vi "HandleStopAsync.vi"(8 "error in (no error)":errorcluster, 11 "S4GUI in":refnum<class "S4GUI.lvclass">) -> (0 "error out":errorcluster, 3 "S4GUI out":refnum<class "S4GUI.lvclass">)   [LabVIEW 2018, in "S4GUI.lvclass"]
uses:
  S4GUI.lvclass
  S4GUI.lvclass/S4GUI.ctl
  Instrument/Instrument.lvclass/Instrument.ctl
  Instrument/Instrument.lvclass
  Device/Optics/Opt_Selector/Opt_Selector.lvclass
  Acquisition/Acquisition.lvclass
  StateMachine/State Machine.lvclass
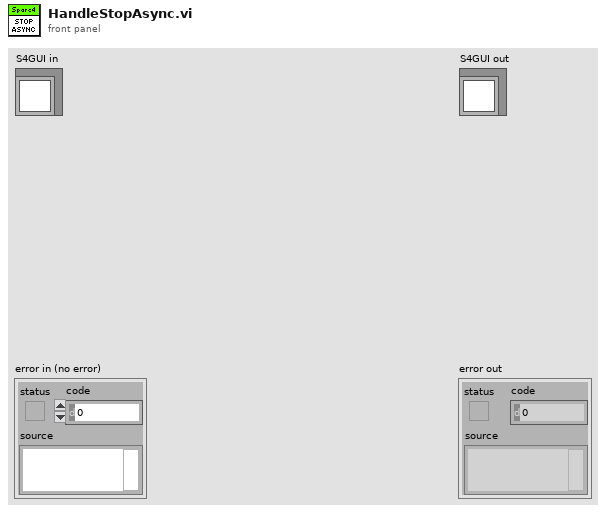
[diagram p1: front panel]
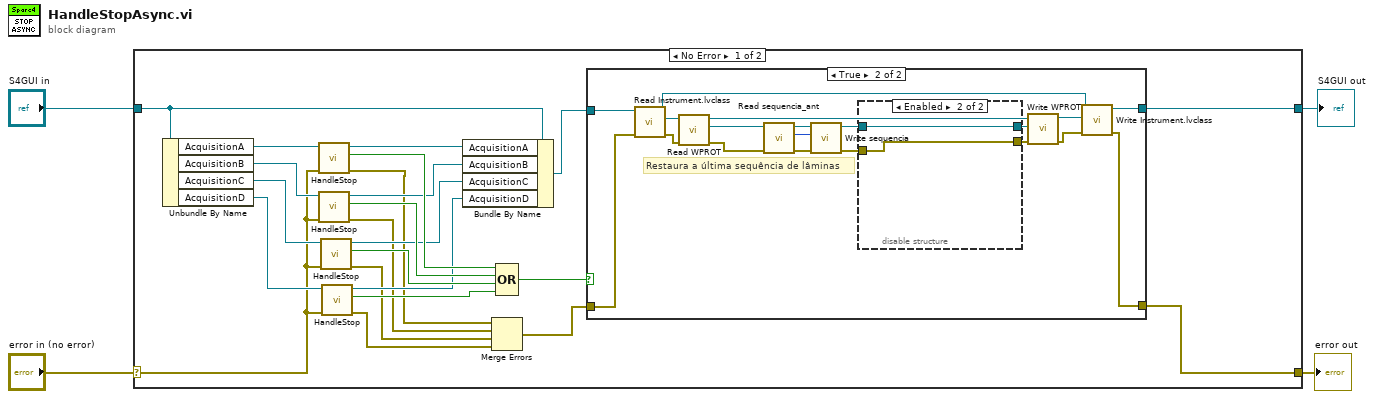
[diagram p0: block diagram]
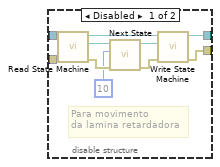
[diagram p3: hidden frame]
diagram:
  n1 = case shown="No Error" "error in (no error)" {
    selector: "error in (no error)" -> [w10 w62]
    tunnel: [w27 w62] -> w3
    tunnel: [w26 w61] -> w1
    tunnel: "S4GUI in" -> [w16 w61]
    frame No Error {
      n2 = Unbundle By Name(w16) -> ("AcquisitionA"=w25:refnum<class "Acquisition.lvclass">, "AcquisitionB"=w24:refnum<class "Acquisition.lvclass">, "AcquisitionC"=w23:refnum<class "Acquisition.lvclass">, "AcquisitionD"=w22:refnum<class "Acquisition.lvclass">)
      n3 = call-dynamic "HandleStop.vi"("error in (no error)"=w10, "Acquisition in"=w25) -> ("error out"=w9:errorcluster, "stop?"=w21:bool, "Acquisition out"=w14:refnum<class "Acquisition.lvclass">)  [unwired: 7 in]
      n4 = call-dynamic "HandleStop.vi"("error in (no error)"=w10, "Acquisition in"=w24) -> ("error out"=w8:errorcluster, "stop?"=w20:bool, "Acquisition out"=w13:refnum<class "Acquisition.lvclass">)  [unwired: 7 in]
      n5 = call-dynamic "HandleStop.vi"("error in (no error)"=w10, "Acquisition in"=w23) -> ("error out"=w7:errorcluster, "stop?"=w19:bool, "Acquisition out"=w12:refnum<class "Acquisition.lvclass">)  [unwired: 7 in]
      n6 = call-dynamic "HandleStop.vi"("error in (no error)"=w10, "Acquisition in"=w22) -> ("error out"=w6:errorcluster, "stop?"=w18:bool, "Acquisition out"=w11:refnum<class "Acquisition.lvclass">)  [unwired: 7 in]
      n7 = Bundle By Name(cluster=w16, "AcquisitionA"=w14, "AcquisitionB"=w13, "AcquisitionC"=w12, "AcquisitionD"=w11) -> (w15:refnum<class "S4GUI.lvclass">)
      n8 = Merge Errors(w9, w8, w7, w6) -> (w5:errorcluster)
      n9 = Compound Arithmetic op=OR(w21, w20, w19, w18) -> (w17:bool)
      n10 = case shown="True" w17 {
        tunnel: w15 -> [w29 w31]
        tunnel: w5 -> [w28 w30]
        tunnel: [w28 w33] -> w27
        tunnel: [w29 w32] -> w26
        frame False {
        }
        frame True {
          # "Restaura a última sequência de lâminas"
          n11 = call "Read Instrument.lvclass.vi"("error in (no error)"=w30, "S4ACS_GUI in"=w31) -> ("error out"=w38:errorcluster, "Instrument.lvclass"=w35:refnum<class "Instrument.lvclass">, "S4ACS_GUI out"=w34:refnum<class "S4GUI.lvclass">)  [unwired: 7 in]
          n12 = call "Read WPROT.vi"("error in (no error)"=w38, "Instrument in"=w35) -> ("error out"=w39:errorcluster, "Opt_Selector.lvclass"=w37:refnum<class "Opt_Selector.lvclass">, "Instrument out"=w36:refnum<class "Instrument.lvclass">)  [unwired: 7 in]
          n13 = call-dynamic "Read sequencia_ant.vi"("error in (no error)"=w39, "Opt_Selector in"=w37) -> ("error out"=w43:errorcluster, "sequencia_ant"=w44:u16, "Opt_Selector out"=w42:refnum<class "Opt_Selector.lvclass">)  [unwired: 7 in]
          n14 = call-dynamic "Write sequencia.vi"("error in (no error)"=w43, "sequencia"=w44, "Opt_Selector in"=w42) -> ("error out"=w46:errorcluster, "Opt_Selector out"=w45:refnum<class "Opt_Selector.lvclass">)  [unwired: 7 in]
          n15 = disable-structure shown="Enabled" {
            disable-tunnel: [w58 w59] -> w48
            disable-tunnel: [w57 w60] -> w47
            disable-tunnel: w46 -> [w55 w59]
            disable-tunnel: w45 -> [w54 w60]
            frame Disabled {
              # "Para movimento \nda lamina retardadora"
              n16 = call-dynamic "Read State Machine.vi"("error in (no error)"=w55, "Device in"=w54) -> ("error out"=w52:errorcluster, "State Machine.lvclass"=w50:refnum<class "State Machine.lvclass">, "Device out"=w56:refnum<class "Opt_Selector.lvclass">)  [unwired: 7 in]
              n17 = call "Next State.vi"("error in (no error)"=w52, "New_State"=10, "State Machine in"=w50) -> ("error out"=w53:errorcluster, "State Machine out"=w51:refnum<class "State Machine.lvclass">)  [unwired: 7 in]
              n18 = call-dynamic "Write State Machine.vi"("error in (no error)"=w53, "State Machine.lvclass"=w51, "Device in"=w56) -> ("error out"=w58:errorcluster, "Device out"=w57:refnum<class "Opt_Selector.lvclass">)  [unwired: 7 in]
            }
            frame Enabled {
            }
          }
          n19 = call "Write WPROT.vi"("error in (no error)"=w48, "Opt_Selector.lvclass"=w47, "Instrument in"=w36) -> ("error out"=w40:errorcluster, "Instrument out"=w41:refnum<class "Instrument.lvclass">)  [unwired: 7 in]
          n20 = call "Write Instrument.lvclass.vi"("error in (no error)"=w40, "Instrument.lvclass"=w41, "S4ACS_GUI in"=w34) -> ("error out"=w33:errorcluster, "S4ACS_GUI out"=w32:refnum<class "S4GUI.lvclass">)  [unwired: 7 in]
        }
      }
    }
    frame Error {
    }
  }
  "error out" <- w3
  "S4GUI out" <- w1
